vi "Move Video Window.vi"(9 "Action":T1, 10 "This VI":refnum<vi>, 11 "Poaition Control Ref":refnum<vi>) -> ()   [LabVIEW 2017]
uses:
  <vilib>/Utility/miscctls.llb/LVBoundsTypeDef.ctl
  <vilib>/Utility/miscctls.llb/LVPointTypeDef.ctl
  Video Command type.ctl
  VideoWindowsCommand.ctl
  ABB global.vi
panel:
  out "Screen Coordinates":T2
  out "Bounds":T3
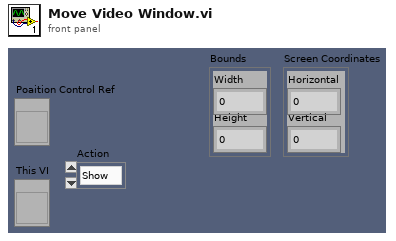
[diagram p1: front panel]
types:
  T1 = typedef "Video Command type.ctl" = enum16{"Show", "Hide", "Exit", "Kick"}
  T2 = typedef "LVPointTypeDef.ctl" = cluster{"Horizontal":i16, "Vertical":i16}
  T3 = typedef "LVBoundsTypeDef.ctl" = cluster{"Width":u32, "Height":u32}
  T4 = typedef "VideoWindowsCommand.ctl" = cluster{"Position":cluster{"Right":i32, "Bottom":i32}, "Action":T1, "Camera Addresses":cluster{"Camera 1":string, "Camera 2":string, "Mobile":string}}
  T5 = cluster{"Camera 1":string, "Camera 2":string, "Mobile":string}
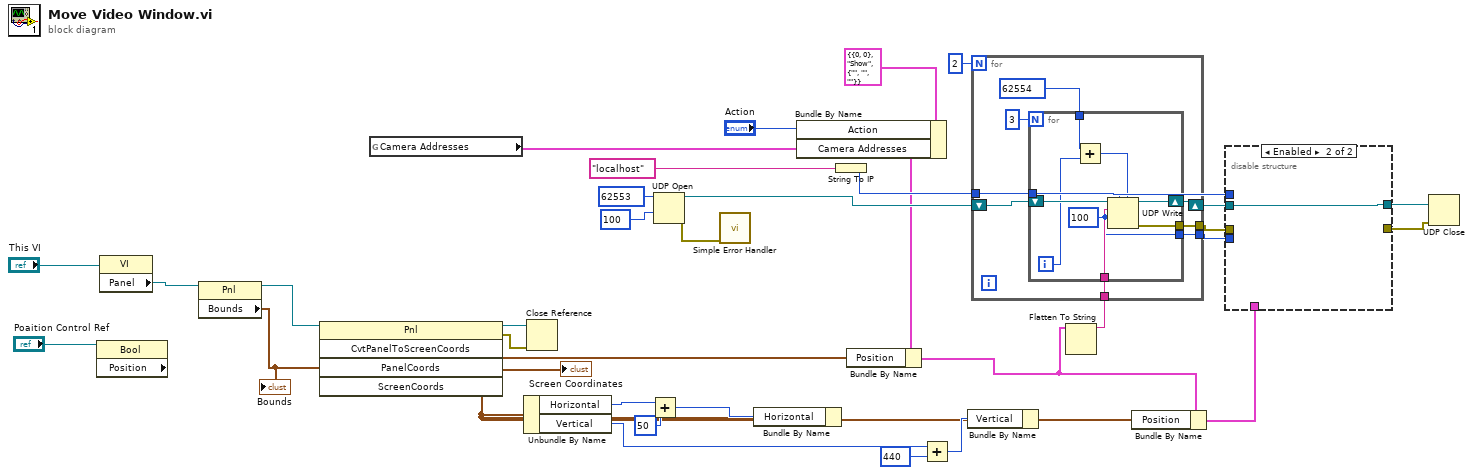
[diagram p0: block diagram]
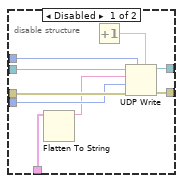
[diagram p2: hidden frame]
diagram:
  n1 = property class="Bool" props=["Position"](reference="Poaition Control Ref") -> ()  [unwired: 1 in, 3 out]
  n2 = property class="VI"(reference="This VI") -> ("Panel"=w31:refnum<vi>)  [unwired: 1 in, 2 out]
  n3 = property class="Pnl"(reference=w31) -> (reference out=w9:refnum<vi>, "Bounds"=w8:T3)  [unwired: 1 in, 1 out]
  "Bounds" <- w8
  n4 = invoke class="Pnl" method="CvtPanelToScreenCoords"(reference=w9, "PanelCoords"=w8) -> (reference out=w33:refnum<vi>, error out=w32:errorcluster, "ScreenCoords"=w7:T2)  [unwired: 3 in, 2 out]
  "Screen Coordinates" <- w7
  n5 = global read "ABB global.vi" "Camera Addresses"() -> (w1:T5)
  n6 = Unbundle By Name(w7) -> ("Horizontal"=w23:i16, "Vertical"=w15:i16)
  n7 = Close Reference(reference=w33, error in (no error)=w32) -> ()  [unwired: 1 out]
  n8 = Add(x=w23, y=i16 50) -> (x+y=w21:i16)
  n9 = UDP Open(9:100 ("timeout ms (25000)"), 11:u16 62553 ("port")) -> (port=w26:refnum<k16>, 0:w6:errorcluster)  [unwired: 3 in, 1 out]
  n10 = call <vilib>:"Simple Error Handler.vi"("error in (no error)"=w6) -> ()  [unwired: 4 in, 5 out]
  n11 = Bundle By Name(cluster=w7, "Horizontal"=w21) -> ()  [unwired: 1 out]
  n12 = Bundle By Name(cluster=T4 {"Position"={"Right"=0, "Bottom"=0}, "Action"=enum."Show", "Camera Addresses"={"Camera 1"="", "Camera 2"="", "Mobile"=""}} ("Cluster"), "Action"="Action", "Camera Addresses"=w1) -> (w4:T4)
  n13 = String To IP(1:"localhost" ("name")) -> (0:w10:u32)
  n14 = Bundle By Name(cluster=w4, "Position"=w7) -> (w12:T4)
  n15 = Add(x=w15, y=i16 440) -> (x+y=w13:i16)
  n16 = Bundle By Name(cluster=w7, "Vertical"=w13) -> ()  [unwired: 1 out]
  n17 = Flatten To String(anything=w12) -> (data string=w28:string)  [unwired: 3 in, 2 out]
  n18 = for {
    N: 2 -> [_]
    tunnel: w28 -> [w41]
    tunnel: [w39] -> w20
    tunnel: [w37] -> w16
    tunnel: w10 -> [w36]
    shift-right: [w38] -> w19
    shift-left: w26 -> [w40]
    n19 = for {
      N: 3 -> [_]
      tunnel: w41 -> [w50]
      tunnel: [w48] -> w39
      tunnel: [w46] -> w37
      tunnel: w36 -> [w45]
      shift-right: [w47] -> w38
      shift-left: w40 -> [w49]
      tunnel: u16 62554 ("port or service name") -> [w43]
      i -> [w44]
      w46 = 100 ("timeout ms (25000)")
      n20 = Add(x=w43, y=w44) -> (x+y=w42:i32)
      n21 = UDP Write(address=w45, port or service name=w42, connection ID=w49, data in=w50, 9:w46) -> (error out=w48:errorcluster, 3:w47:refnum<k16>)  [unwired: 1 in]
    }
  }
  n22 = Bundle By Name(cluster=w12, "Position"=w7) -> (w11:T4)
  n23 = disable-structure shown="Enabled" {
    disable-tunnel: w20 -> [w60 _]
    disable-tunnel: w19 -> [w59 w61]
    disable-tunnel: [w58 w61] -> w18
    disable-tunnel: [w57 _] -> w17
    disable-tunnel: w16 -> [w56 _]
    disable-tunnel: w11 -> [w55 _]
    disable-tunnel: w10 -> [w52 _]
    frame Disabled {
      n24 = Flatten To String(anything=w55) -> (data string=w54:string)  [unwired: 3 in, 2 out]
      n25 = Increment() -> (x=w51:dbl, x+1=w53:dbl)
      n26 = UDP Write(address=w52, port or service name=w53, connection ID=w59, data in=w54, 8:w60, 9:w56) -> (error out=w57:errorcluster, 3:w58:refnum<k16>)
    }
    frame Enabled {
    }
  }
  n27 = UDP Close(connection ID=w18, 8:w17) -> ()  [unwired: 2 out]
